vi "heterochromaticFlicker.vi"() -> ()   [LabVIEW 2009]
uses:
  <vilib>/LabVIEW Interface for Arduino/LabVIEW Interface for Arduino.lvlib
  <vilib>/LabVIEW Interface for Arduino/Type Defs/Pin Mode.ctl
panel:
  in  "Stop":bool
  out "Debug \ninner i\n(which of the\nlights to be flashed)":i32
  out "Debug \nouter i\n(how many \ncycles passed)":i32
  in  "Pin 410nm 2":u8 min=1 max=15 step=1
  in  "Duty Cycle 410nm 3":u8(slide) step=1
  in  "Pin 560nm":u8 min=1 max=15 step=1
  in  "Pin 410nm":u8 min=1 max=15 step=1
  out "Flicker period [ms]":dbl
  in  "Flicker Freq [Hz]":dbl min=0.2 max=100.0 step=0.1
  in  "Duty Cycle 410nm":u8(slide) step=1
  in  "Duty Cycle 560nm":u8(slide) step=1
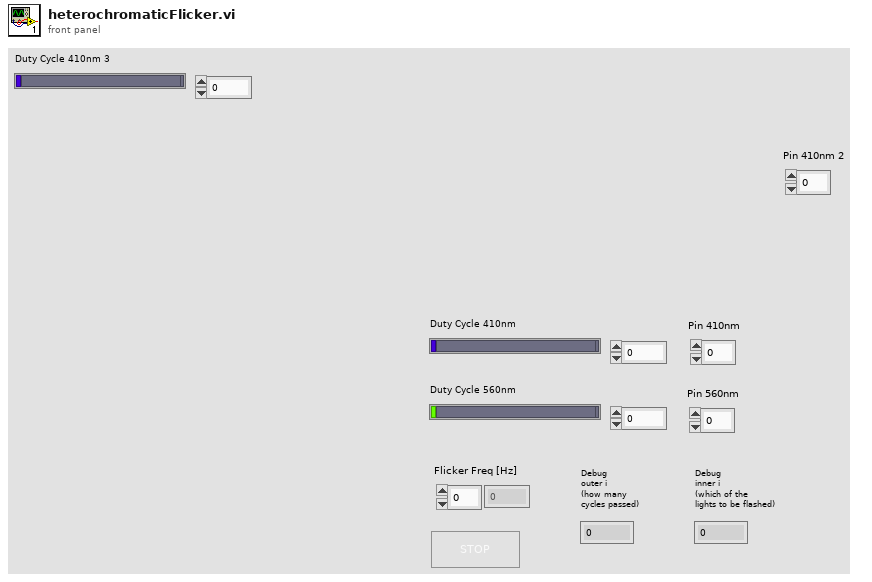
[diagram p1: front panel]
types:
  T1 = typedef "LabVIEW Interface for Arduino.lvlib/Arduino Resource.ctl" = cluster{"VISA resource":refnum<visa-resource-name>, "Board Type":T2, "Connection Type":enum8{"USB / Serial"}, "Bytes Per Packet (15)":u8}
  T2 = typedef "LabVIEW Interface for Arduino.lvlib/Board Type.ctl" = enum16{"Uno", "Dimuelanove w/Atmega 328", "Mega 2560"}
  T3 = typedef "LabVIEW Interface for Arduino.lvlib/Pin Mode.ctl" = enum8{"Input", "Output"}
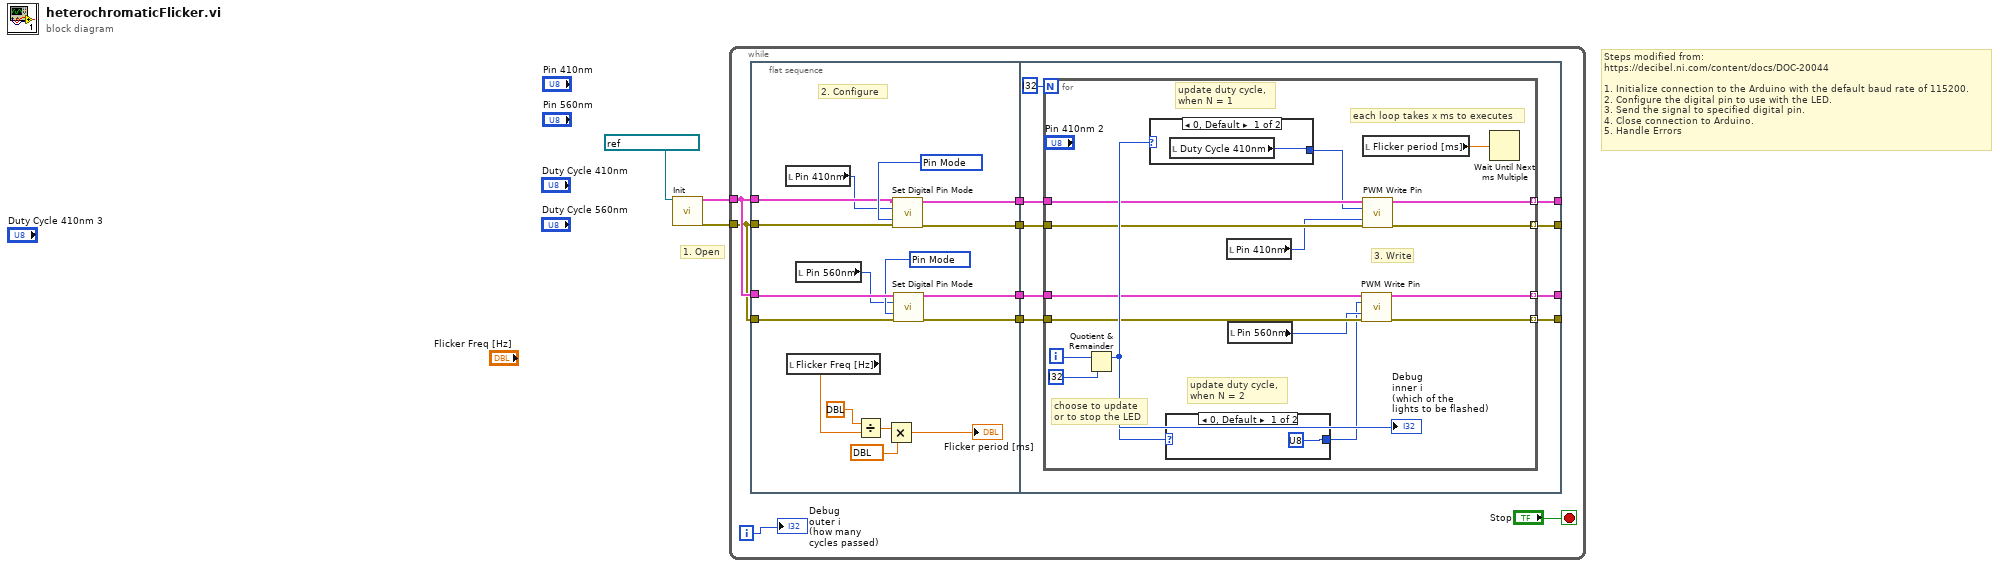
[diagram p0: block diagram]
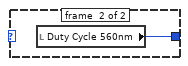
[diagram p2: hidden frame]
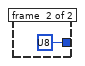
[diagram p3: hidden frame]
diagram:
  # "1. Open"
  # "Steps modified from:\nhttps://decibel.ni.com/content/docs/DOC-20044\n\n1. Initialize connection to the Arduino with the default baud rate of 115200.\n2. Configure the digital pin to use with the LED.\n3. Send the signal to specified digital pin.\n4. Close connection to Arduino.\n5. Handle Errors"
  n1 = call <vilib>:"Init.vi"("VISA resource"=refnum<visa-resource-name> ?) -> ("Arduino Resource"=w3:T1, "error out"=w2:errorcluster)  [unwired: 17 in]
  n2 = while {
    tunnel: w3 -> [w5]
    tunnel: w2 -> [w4]
    i -> [w6]
    stop <- "Stop" stop-if-true
    n3 = flat-sequence {
      tunnel: w5 -> [w27]
      tunnel: w4 -> [w26]
      tunnel: w5 -> [w25]
      tunnel: w4 -> [w24]
      tunnel: [w20] -> w11
      tunnel: [w19] -> w10
      tunnel: [w18] -> w9
      tunnel: [w17] -> w8
      tunnel: w11 -> [w36]
      tunnel: w10 -> [w35]
      tunnel: w9 -> [w34]
      tunnel: w8 -> [w33]
      tunnel: [w32] -> _
      tunnel: [w31] -> _
      tunnel: [w30] -> _
      tunnel: [w29] -> _
      frame #0 {
        # "2. Configure"
        n4 = local read "Pin 410nm"() -> (w21:u8)
        n5 = local read "Flicker Freq [Hz]"() -> (w12:dbl)
        n6 = local read "Pin 560nm"() -> (w22:u8)
        n7 = Divide(x=dbl ?, y=w12) -> (x/y=w14:dbl)
        n8 = Multiply(x=w14, y=dbl ?) -> (x*y=→"Flicker period [ms]":dbl)
        n9 = call <vilib>:"Set Digital Pin Mode.vi"("Arduino Resource"=w27, "Digital I/O Pin"=w21, "Pin Mode (Input)"=T3 ?, "error in"=w26) -> ("Arduino Resource"=w18:T1, "error out"=w17:errorcluster)  [unwired: 10 in]
        n10 = call <vilib>:"Set Digital Pin Mode.vi"("Arduino Resource"=w25, "Digital I/O Pin"=w22, "Pin Mode (Input)"=T3 ?, "error in"=w24) -> ("Arduino Resource"=w20:T1, "error out"=w19:errorcluster)  [unwired: 10 in]
      }
      frame #1 {
        n11 = for {
          N: i32 ? -> [_]
          tunnel: w36 -> [w49]
          tunnel: w35 -> [w48]
          tunnel: w34 -> [w47]
          tunnel: w33 -> [w46]
          tunnel: [w45] -> w29 mode=indexing
          tunnel: [w44] -> w32 mode=indexing
          tunnel: [w43] -> w31 mode=indexing
          tunnel: [w42] -> w30 mode=indexing
          i -> [w51]
          # "update duty cycle, \nwhen N = 2"
          # "update duty cycle, \nwhen N = 1"
          # "each loop takes x ms to executes"
          # "3. Write"
          # "choose to update \nor to stop the LED"
          n12 = Quotient & Remainder(x=w51, y=i32 ?) -> (x-y*floor(x/y)=w50:i32)  [unwired: 1 out]
          n13 = case shown="0, Default" w50 {
            tunnel: [w56 u8 ? ("Duty Cycle")] -> w38
            frame #0 {
              n14 = local read "Duty Cycle 410nm"() -> (w56:u8)
            }
            frame #1 {
            }
          }
          n15 = case shown="0, Default" w50 {
            tunnel: [u8 ? ("Duty Cycle") w55] -> w40
            frame #0 {
            }
            frame #1 {
              n16 = local read "Duty Cycle 560nm"() -> (w55:u8)
            }
          }
          n17 = local read "Pin 410nm"() -> (w39:u8)
          n18 = local read "Pin 560nm"() -> (w41:u8)
          n19 = call <vilib>:"PWM Write Pin.vi"("Arduino Resource"=w49, "Duty Cycle (0 - 255)"=w40, "PWM Pin (3)"=w41, "error in"=w48) -> ("Arduino Resource"=w44:T1, "error out"=w43:errorcluster)  [unwired: 10 in]
          n20 = local read "Flicker period [ms]"() -> (w53:dbl)
          n21 = call <vilib>:"PWM Write Pin.vi"("Arduino Resource"=w47, "Duty Cycle (0 - 255)"=w38, "PWM Pin (3)"=w39, "error in"=w46) -> ("Arduino Resource"=w45:T1, "error out"=w42:errorcluster)  [unwired: 10 in]
          n22 = Wait Until Next ms Multiple(millisecond multiple=w53) -> ()  [unwired: 1 out]
          "Debug \ninner i\n(which of the\nlights to be flashed)" <- w51
        }
      }
    }
    "Debug \nouter i\n(how many \ncycles passed)" <- w6
  }
